vi "Autonomous Independent.vi"   [LabVIEW 2016]
doc: "This VI is called when autonomous begins, and will automatically be terminated when autonomous ends. You can carry out timed or sensor driven robot movement independently without needing to return to the caller."
uses:
  <vilib>/Rock Robotics/WPI/Utilities/WPI_GetSetVariantRefNum.vi
  <vilib>/Rock Robotics/Network Tables/NT Read String.vi
  <vilib>/Rock Robotics/Network Tables/NT Write Numeric Array.vi
panel:
  # "Be sure to right-click and choose Data Operations>>Make Current Value default if you want to save the array values with the VI"
types:
  T1 = typedef "WPI_JoystickDevRef.ctl" = cluster{"Device":T2}
  T2 = typedef "WPI_JoystickDeviceEnum.ctl" = enum16{"USB 0", "USB 1", "USB 2", "USB 3", "USB 4", "USB 5"}
  T3 = typedef "WPI_MotorControlDeviceRef.ctl" = cluster{"DeviceStatus":errorcluster, "Type":T4, "PWM":cluster{"PWM Channel":T5, "DeadBand":T6}, "CAN":cluster{"Device Number":u8, "SetOutput VI Ref":variant, "GetOutput VI Ref":variant, "Enable VI Ref":variant, "Disable VI Ref":variant, "Data":variant}, "Invert":bool}
  T4 = typedef "WPI_MotorControlType.ctl" = enum16{"PWM", "CAN"}
  T5 = typedef "FPGA_DIOPWMChannel.ctl" = enum8{"PWM 0", "PWM 1", "PWM 2", "PWM 3", "PWM 4", "PWM 5", "PWM 6", "PWM 7", "PWM 8", "PWM 9", "PWM MXP 0", "PWM MXP 1", "PWM MXP 2", "PWM MXP 3", "PWM MXP 4", "PWM MXP 5", "PWM MXP 6", "PWM MXP 7", "PWM MXP 8", "PWM MXP 9", "Invalid"}
  T6 = typedef "WPI_PWMDeadband.ctl" = cluster{"Name":string, "maxPositivePwm":i32, "minPositivePwm":i32, "centerPwm":i32, "maxNegativePwm":i32, "minNegativePwm":i32, "angularRange":u16}
  T7 = cluster{"MotorControlDevRef":T3, "MotorControlDevRef":T3}
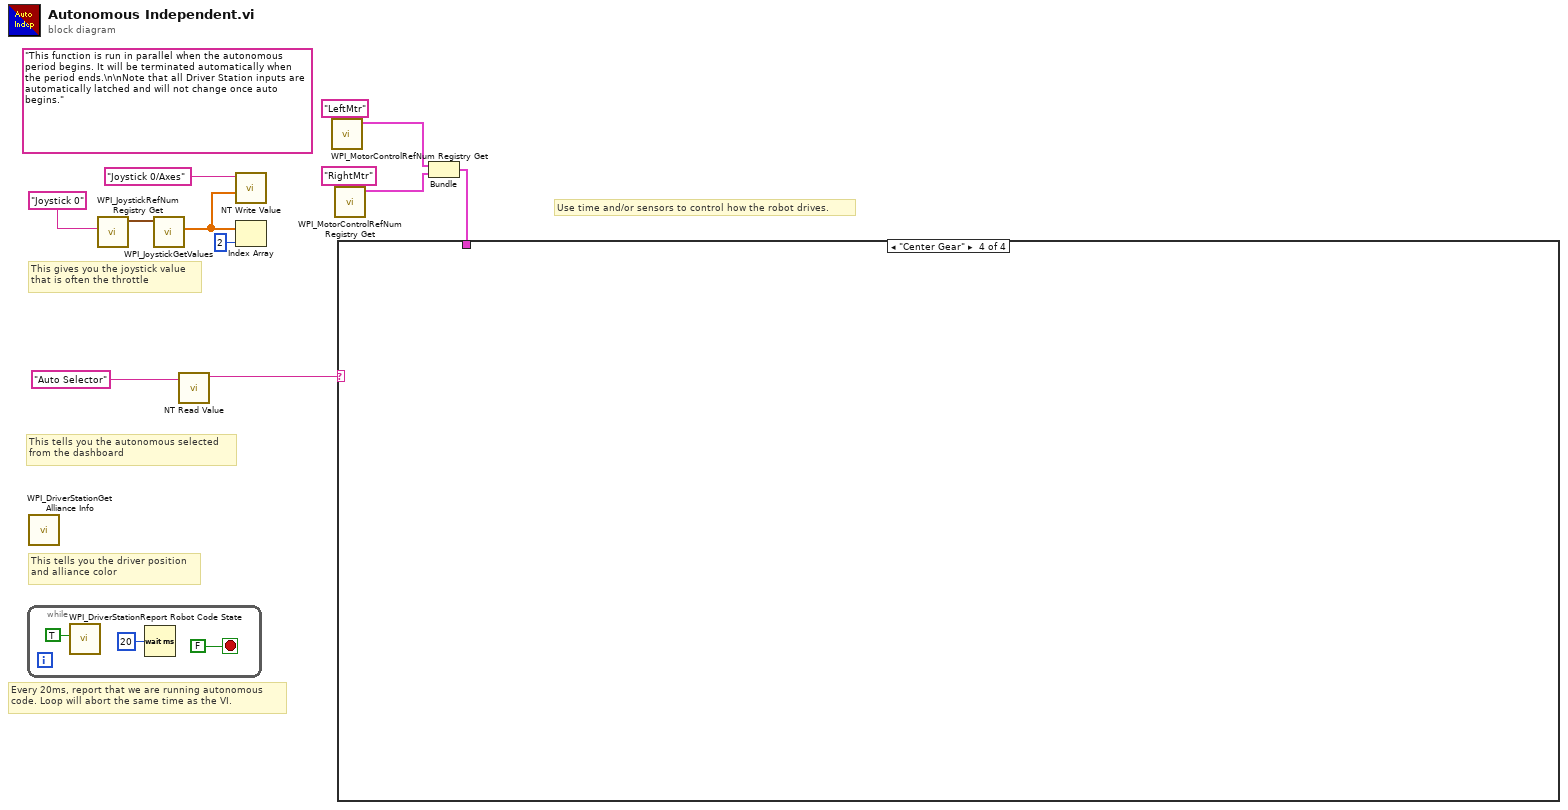
[diagram p0: block diagram]
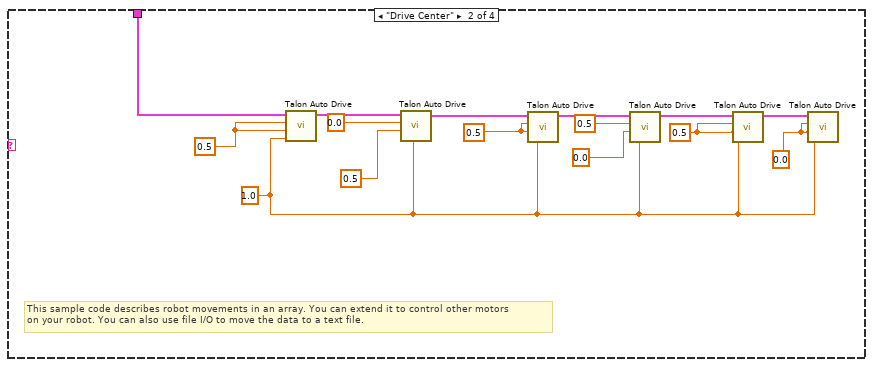
[diagram p3: hidden frame]
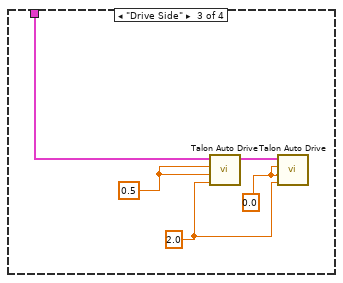
[diagram p4: hidden frame]
diagram:
  (unwired) "This function is run in parallel when the autonomous period begins. It will be terminated automatically when the period ends.\n\nNote that all Driver Station inputs are automatically latched and will not change once auto begins."
  # "This tells you the autonomous selected\nfrom the dashboard"
  # "Every 20ms, report that we are running autonomous\ncode. Loop will abort the same time as the VI."
  # "This gives you the joystick value\nthat is often the throttle"
  # "Use time and/or sensors to control how the robot drives."
  # "This tells you the driver position\nand alliance color"
  n1 = while {
    stop <- FALSE stop-if-true
    n2 = call <vilib>:"WPI_DriverStationReport Robot Code State.vi"("Autonomous"=TRUE) -> ()  [unwired: 10 in, 1 out]
    n3 = Wait (ms)(milliseconds to wait=u32 20) -> ()  [unwired: 1 out]
  }
  n4 = call <vilib>:"WPI_DriverStationGet Alliance Info.vi"() -> ()  [unwired: 12 out]
  n5 = call <vilib>:"WPI_JoystickRefNum Registry Get.vi"("refnum name"="Joystick 0") -> ("JoystickDevRef"=w11:T1)  [unwired: 1 in, 9 out]
  n6 = call <vilib>:"WPI_JoystickGetValues.vi"("JoystickDevRef"=w11) -> ("Axes"=w7:dbl[])  [unwired: 6 in, 4 out]
  n7 = call-poly <vilib>:"NT Read Value.vi"("Name"="Auto Selector") -> ("String"=w8:string)  [unwired: 9 in, 1 out]
  n8 = call-poly <vilib>:"NT Write Value.vi"("Numeric Array"=w7, "Name"="Joystick 0/Axes") -> ()  [unwired: 9 in, 1 out]
  n9 = Index Array(array=w7, index=2) -> ()  [unwired: 1 out]
  n10 = call <vilib>:"WPI_MotorControlRefNum Registry Get.vi"("refnum name"="LeftMtr") -> ("MotorControlDevRef"=w4:T3)  [unwired: 9 in, 1 out]
  n11 = call <vilib>:"WPI_MotorControlRefNum Registry Get.vi"("refnum name"="RightMtr") -> ("MotorControlDevRef"=w5:T3)  [unwired: 9 in, 1 out]
  n12 = Bundle("MotorControlDevRef"=w4, "MotorControlDevRef"=w5) -> (w1:T7)  [unwired: 1 in]
  n13 = case shown="\"Center Gear\"" w8 {
    tunnel: w1 -> [_ w22 w34 _]
    frame Default {
      # "You can put your main auto here, or you can right-click on the case and make any\nother frame be the default case."
      # "This is the frame that will execute if no selection is made, or if it is not recognized"
    }
    frame "Drive Center" {
      w17 = 0.5 ("Right")
      w21 = 0.0 ("Right")
      w23 = 0.5 ("Right")
      w30 = 0.5 ("Right")
      w16 = 1.0 ("Delay (s)")
      # "This sample code describes robot movements in an array. You can extend it to control other motors\non your robot. You can also use file I/O to move the data to a text file."
      n14 = call "Talon Auto Drive.vi"("Delay (s)"=w16, "Right"=w30, "Left"=w30, "Cluster"=w22) -> ("output cluster"=w29:T7)  [unwired: 7 in]
      n15 = call "Talon Auto Drive.vi"("Delay (s)"=w16, "Right"=0.5, "Left"=0.0, "Cluster"=w29) -> ("output cluster"=w19:T7)  [unwired: 7 in]
      n16 = call "Talon Auto Drive.vi"("Delay (s)"=w16, "Right"=w17, "Left"=w17, "Cluster"=w19) -> ("output cluster"=w18:T7)  [unwired: 7 in]
      n17 = call "Talon Auto Drive.vi"("Delay (s)"=w16, "Right"=0.0 ("Left"), "Left"=0.5 ("Right"), "Cluster"=w18) -> ("output cluster"=w24:T7)  [unwired: 7 in]
      n18 = call "Talon Auto Drive.vi"("Delay (s)"=w16, "Right"=w23, "Left"=w23, "Cluster"=w24) -> ("output cluster"=w20:T7)  [unwired: 7 in]
      n19 = call "Talon Auto Drive.vi"("Delay (s)"=w16, "Right"=w21, "Left"=w21, "Cluster"=w20) -> ()  [unwired: 7 in, 1 out]
    }
    frame "Drive Side" {
      w33 = 0.0 ("Right")
      w35 = 0.5 ("Right")
      w31 = 2.0 ("Delay (s)")
      n20 = call "Talon Auto Drive.vi"("Delay (s)"=w31, "Right"=w35, "Left"=w35, "Cluster"=w34) -> ("output cluster"=w32:T7)  [unwired: 7 in]
      n21 = call "Talon Auto Drive.vi"("Delay (s)"=w31, "Right"=w33, "Left"=w33, "Cluster"=w32) -> ()  [unwired: 7 in, 1 out]
    }
    frame "Center Gear" {
    }
  }
